vi "File Size Deletion VI.vi"(9 "Scan Files":bool, 10 "File Size Deletion Threshold (Bytes)":i64, 11 "Folder With Files in Question":path) -> ()   [LabVIEW 2017]
panel:
  in  "Stop":bool
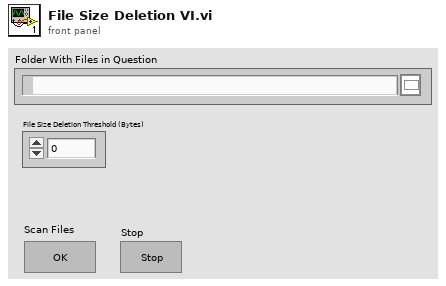
[diagram p1: front panel]
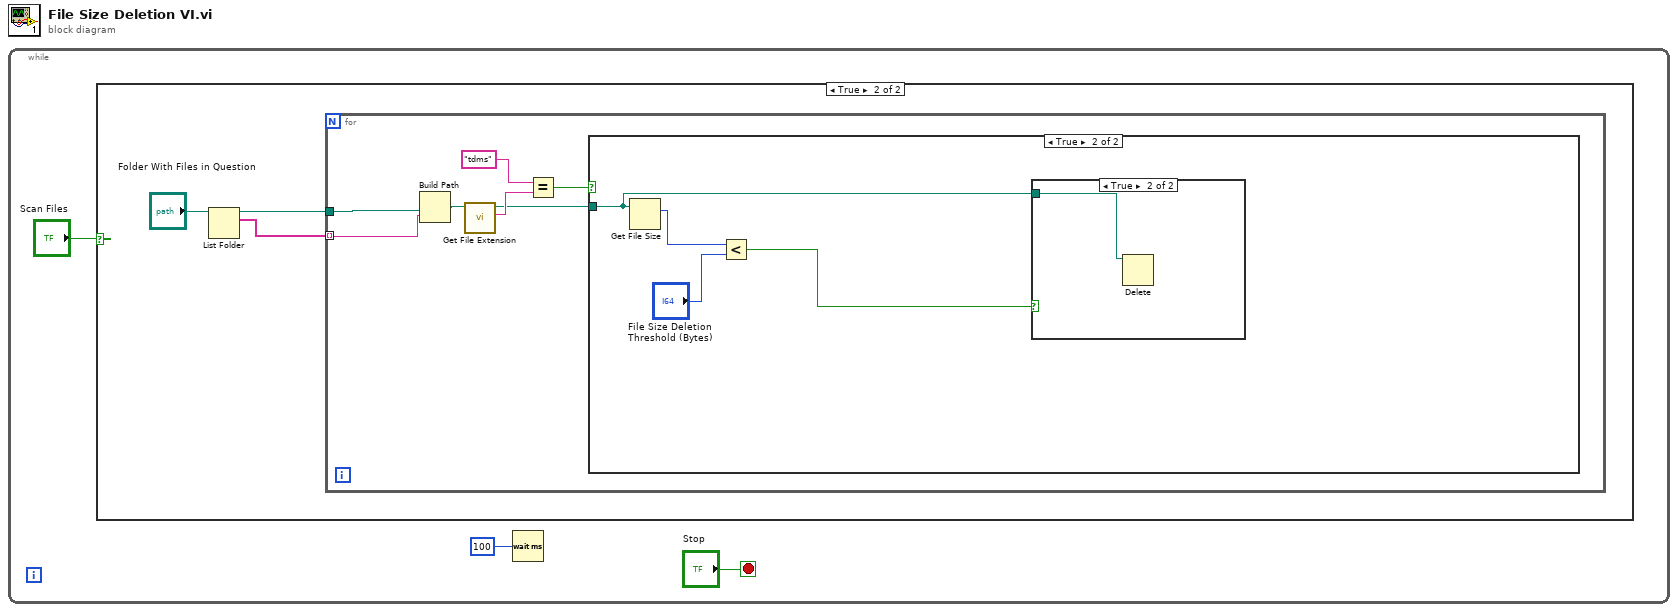
[diagram p0: block diagram]
diagram:
  n1 = while {
    stop <- "Stop" stop-if-true
    n2 = case shown="True" "Scan Files" {
      frame False {
      }
      frame True {
        n3 = List Folder(path="Folder With Files in Question") -> (path out=w4:path, filenames=w5:string[])  [unwired: 3 in, 2 out]
        n4 = for {
          tunnel: w5 -> [w13] mode=indexing
          tunnel: w4 -> [w7]
          n5 = Build Path(base path=w7, name or relative path=w13) -> (appended path=w12:path)
          n6 = call <vilib>:"Get File Extension.vi"("file"=w12) -> ("lowercase file extension"=w11:string, "dup file"=w8:path)  [unwired: 6 in, 3 out]
          n7 = Equal?(x="tdms", y=w11) -> (x = y?=w9:bool)
          n8 = case shown="True" w9 {
            tunnel: w8 -> [_ w14]
            frame False {
            }
            frame True {
              n9 = Get File Size(file=w14) -> (size (in bytes)=w17:i64)  [unwired: 1 in, 2 out]
              n10 = Less?(x=w17, y="File Size Deletion Threshold (Bytes)") -> (x < y?=w15:bool)
              n11 = case shown="True" w15 {
                tunnel: w14 -> [_ w18]
                frame False {
                }
                frame True {
                  n12 = Delete(path (use dialog)=w18) -> ()  [unwired: 4 in, 3 out]
                }
              }
            }
          }
        }
      }
    }
    n13 = Wait (ms)(milliseconds to wait=u32 100 ("millisecond multiple")) -> ()  [unwired: 1 out]
  }
